vi "SLL DE Reorder Virtual Channels Values_Boolean.vi"(8 "error in (no error)":errorcluster, 10 "Channel Order":i32[](array[numeric]), 11 "Disordered DI Data":bool[](array[boolean])) -> (0 "error out":errorcluster, 3 "Ordered DI Data":bool[](array[boolean]))   [LabVIEW 2013]
doc: "Copyright © 2005, Soliton Technologies.\nAll rights reserved."
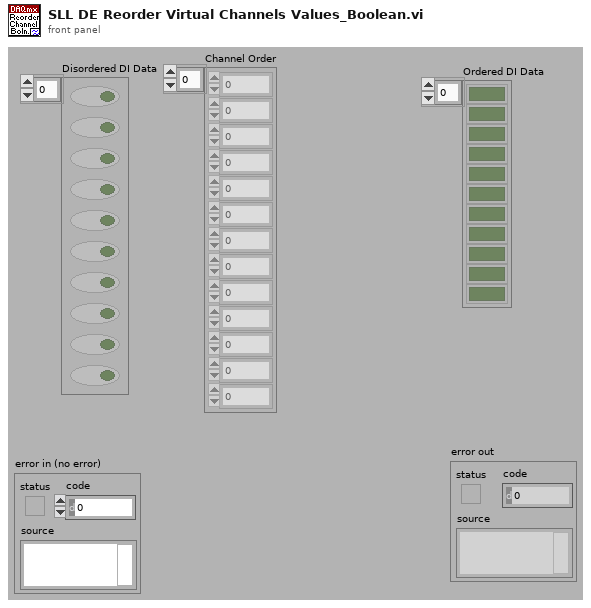
[diagram p1: front panel]
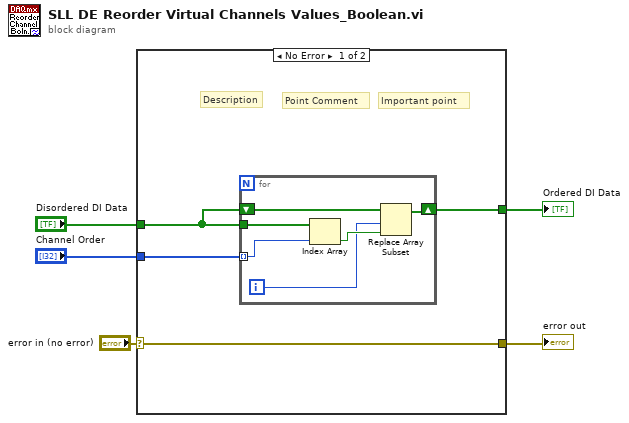
[diagram p0: block diagram]
diagram:
  n1 = case shown="No Error" "error in (no error)" {
    selector: "error in (no error)" -> [w9 w17]
    tunnel: [w9 w17] -> w4
    tunnel: "Disordered DI Data" -> [w8 w16]
    tunnel: "Channel Order" -> [w7 _]
    tunnel: [w6 w16] -> w1
    frame No Error {
      # "Point Comment"
      # "Important point"
      # "Description"
      n2 = for {
        shift-right: [w10] -> w6
        shift-left: w8 -> [w13]
        tunnel: w8 -> [w15]
        tunnel: w7 -> [w14] mode=indexing
        i -> [w11]
        n3 = Index Array(array=w15, index=w14) -> (element=w12:bool)
        n4 = Replace Array Subset(array=w13, new element=w12, index=w11) -> (w10:bool[])
      }
    }
    frame Error {
    }
  }
  "error out" <- w4
  "Ordered DI Data" <- w1
